vi "getTaskChannel.vi"(8 "error in (no error)":errorcluster, 11 "ExampleTask_StopNotifier in":refnum<class "Task_BoolUserEventStopMech.lvclass">) -> (0 "error out":errorcluster, 2 "taskChannek":refnum<class "ITaskChannel.lvclass">, 3 "ExampleTask_StopNotifier out":refnum<class "Task_BoolUserEventStopMech.lvclass">)   [LabVIEW 2023, in "Task_BoolUserEventStopMech.lvclass"]
doc: "Returns the Task Channel type used by the task."
uses:
  Task_BoolUserEventStopMech.lvclass
  ITaskChannel/ITaskChannel.lvclass
  BoolUETaskChannel/BoolUETaskChannel.lvclass
  C:/projects/TLC_Daemon/source/ITaskChannel/ITaskChannel.lvclass
  Task_BoolUserEventStopMech.lvclass/Task_BoolUserEventStopMech.ctl
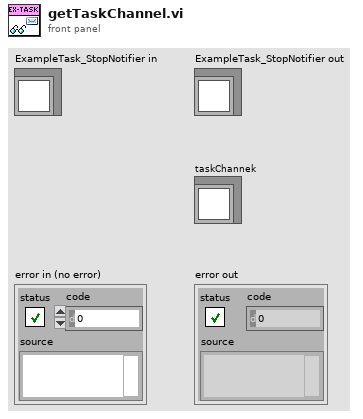
[diagram p1: front panel]
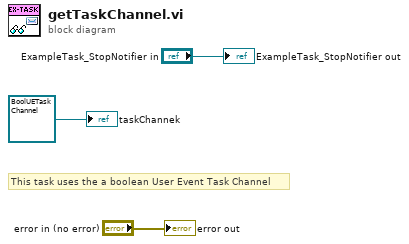
[diagram p0: block diagram]
diagram:
  # "This task uses the a boolean User Event Task Channel"
  "error out" <- "error in (no error)"
  "ExampleTask_StopNotifier out" <- "ExampleTask_StopNotifier in"
  "taskChannek" <- refnum<class "BoolUETaskChannel.lvclass"> refnum ("TLC_Daemon.lvlib:BoolUserEventStopMechanism.lvclass")
